vi "Get Desired Size.vi"(8 "error in (no error)":errorcluster, 11 "Worker Value ArrayPanel in":refnum<class "Value Editor Template.lvclass">) -> (0 "error out":errorcluster, 2 "Desired Size":T1, 3 "Worker Value ArrayPanel out":refnum<class "Value Editor Template.lvclass">)   [LabVIEW 2020, in "Value Editor Template.lvclass"]
uses:
  Value Editor Template.lvclass
  <vilib>/IlluminatedG/IG OOPanel/OOPanel/ArrayPanel/Desired Size.ctl
  Value Editor Template.lvclass/Value Editor Template.ctl
  <vilib>/IlluminatedG/IG OOPanel/OOPanel/OOPanel.lvlib
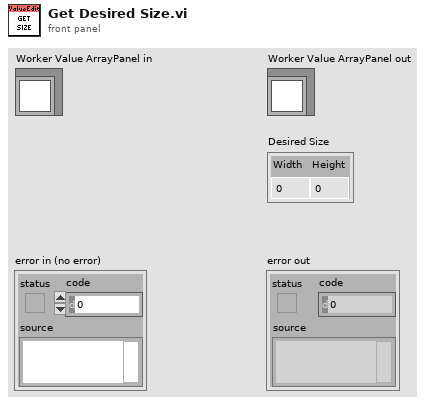
[diagram p1: front panel]
types:
  T1 = typedef "OOPanel.lvlib/Desired Size.ctl" = cluster{"Width":u32, "Height":u32}
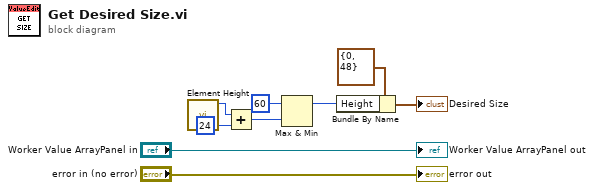
[diagram p0: block diagram]
diagram:
  n1 = call "Element Height.vi"() -> ("Element Height"=w5:i16)  [unwired: 11 in]
  n2 = Add(x=w5, y=i16 24) -> (x+y=w3:i16)
  n3 = Max & Min(x=i16 60, y=w3) -> (max(x,y)=w1:i16)  [unwired: 1 out]
  n4 = Bundle By Name(cluster=T1 {"Width"=0, "Height"=48} ("Desired Size"), "Height"=w1) -> (→"Desired Size":T1)
  "error out" <- "error in (no error)"
  "Worker Value ArrayPanel out" <- "Worker Value ArrayPanel in"
